vi "target - multi rate - variables - fileIO.vi"() -> ()   [LabVIEW 2011]
uses:
  Output - Cluster.ctl
  <vilib>/Platform/TimedLoop/XDataNode/timing_clust.ctl
  <vilib>/Platform/TimedLoop/XDataNode/nitl_modes.ctl
  <vilib>/Platform/TimedLoop/XDataNode/wakeup.ctl
  Input - Cluster.ctl
  <vilib>/functionblocks/Counter/Count Up/Count Up.vi
  <vilib>/functionblocks/Control/PID/PID.vi
  <vilib>/Platform/TimedLoop/XDataNode/XDataNode.xnode
  <vilib>/functionblocks/FB Core/FB Core.xnode
  <vilib>/functionblocks/FB Property/FB Overlay DBL.ctl
  <vilib>/Platform/TimedLoop/XDataNode/XDNodeRunTimeDep.lvlib
  <vilib>/functionblocks/NI_FunctionBlock Libraries.lvlib
panel:
  in  "shiftReg":T1
  in  "Output - Cluster":T2 {"TS-4" format="%#.2g"; "FS-2" format="%.2g"; "FS-1" format="%.2g"}
  # "The Network Variable Engine and Variable Client Support must be installed on the RT target\nfor this application to function properly. If the Network Variable Engine is not supported on\nthe target (e.g.  FP-2000 with <32MB of RAM), open the project and move the variable library\nto My Computer in the project. Doing this will deploy the variables to localhost but\nwill still require that Variable Client Support be installed on the RT target."
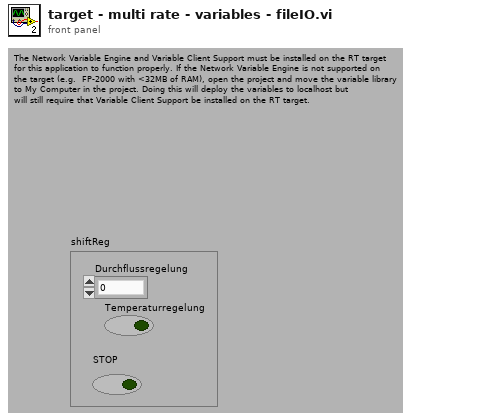
[diagram p1: front panel]
types:
  T1 = cluster{"Durchflussregelung":dbl, "Temperaturregelung":bool, "STOP":bool}
  T2 = typedef "Output - Cluster.ctl" = cluster{"DFS-1 Volumen":u64, "FS-3":dbl, "DFS-1 Durchfluss":dbl, "DS-1":dbl, "V-10 0":bool, "V-14 0":bool, "FS-1":dbl, "FS-2":dbl, "TS-4":dbl, "HS-1":bool, "V-13":u8, "V-15":u8, "P-4 Drehzahl":u8, "P-5 Drehzahl":u8, "Dosierung":bool, "MR Max Füllstand":bool, "MR Min Füllstand":bool, "Dosiermenge":sgl, "V-14 1":bool, "V-10 1":bool, "T-1 Max Füllstand":bool, "T-1 Min Füllstand":bool, "T-2 Max Füllstand":bool, "T-2 Min Füllstand":bool}
  T3 = enum16{"open", "replace", "create", "open or create", "replace or create", "replace or create with confirmation"}
  T4 = typedef "XDNodeRunTimeDep.lvlib/timing_clust.ctl" = cluster{"Expected End [f-1]":u64, "Actual End [f-1]":u64, "Finished Late? [f-1]":bool, "Expected End [i-1]":u64, "Actual End [i-1]":u64, "Finished Late? [i-1]":bool, "Expected Start [i]":u64, "Actual Start [i]":u64, "Expected Start [f]":u64, "Actual Start [f]":u64, "Source Name":string, "Structure Name":string, "Period":i64, "Deadline":i64, "Offset":i64, "Start":i64, "Priority":i32, "Timeout":i32, "Mode":T5, "Wakeup Reason":T6, "Error":errorcluster, "Source Type":string, "Secondary Source Type":string, "Global End Time":u64, "Global Start Time":u64, "Frame Duration":u64, "Iteration Duration":u64, "Assigned CPU":i32, "I/O Scan Engine Mode":u32}
  T5 = typedef "XDNodeRunTimeDep.lvlib/nitl_modes.ctl" = enum32{"No Change", "Process missed periods, maintain original phase", "Discard missed periods, maintain original phase", "Process missed periods, ignore original phase", "Discard missed periods, ignore original phase"}
  T6 = typedef "XDNodeRunTimeDep.lvlib/wakeup.ctl" = enum32{"Normal", "Aborted", "Asynchronous wakeup", "Timing source error", "Timed loop error", "Timeout"}
  T7 = typedef "Input - Cluster.ctl" = cluster{"V-13":u8, "V-15":u8, "Log-Target":bool, "P-4":bool, "P-4 Drehzahl [%]":u8, "Temperaturregelung":bool, "Überdruckregelung":bool, "Füllstandsregulierung":bool, "V-10":bool, "Log-Host":bool, "V-14":bool, "P-5":bool, "P-5 Drehzahl [%]":u8, "HS-1":bool, "Füllstand  P":sgl, "Füllstand I":sgl, "Füllstand D":sgl, "Füllstand Soll [%]":sgl, "Druck  P":sgl, "Druck I":sgl, "Druck D":sgl, "Druck Soll [bar]":sgl, "Temp Soll [°C]":sgl, "Dosierung":bool, "Dosiermenge [l]":sgl, "Dosiergeschw. [l/min]":sgl, "Zulauf":bool, "Hysterese[°C]":sgl, "MR Füllstandsüberwachung":bool, "Zulauf Füllstandsüberwachung":bool}
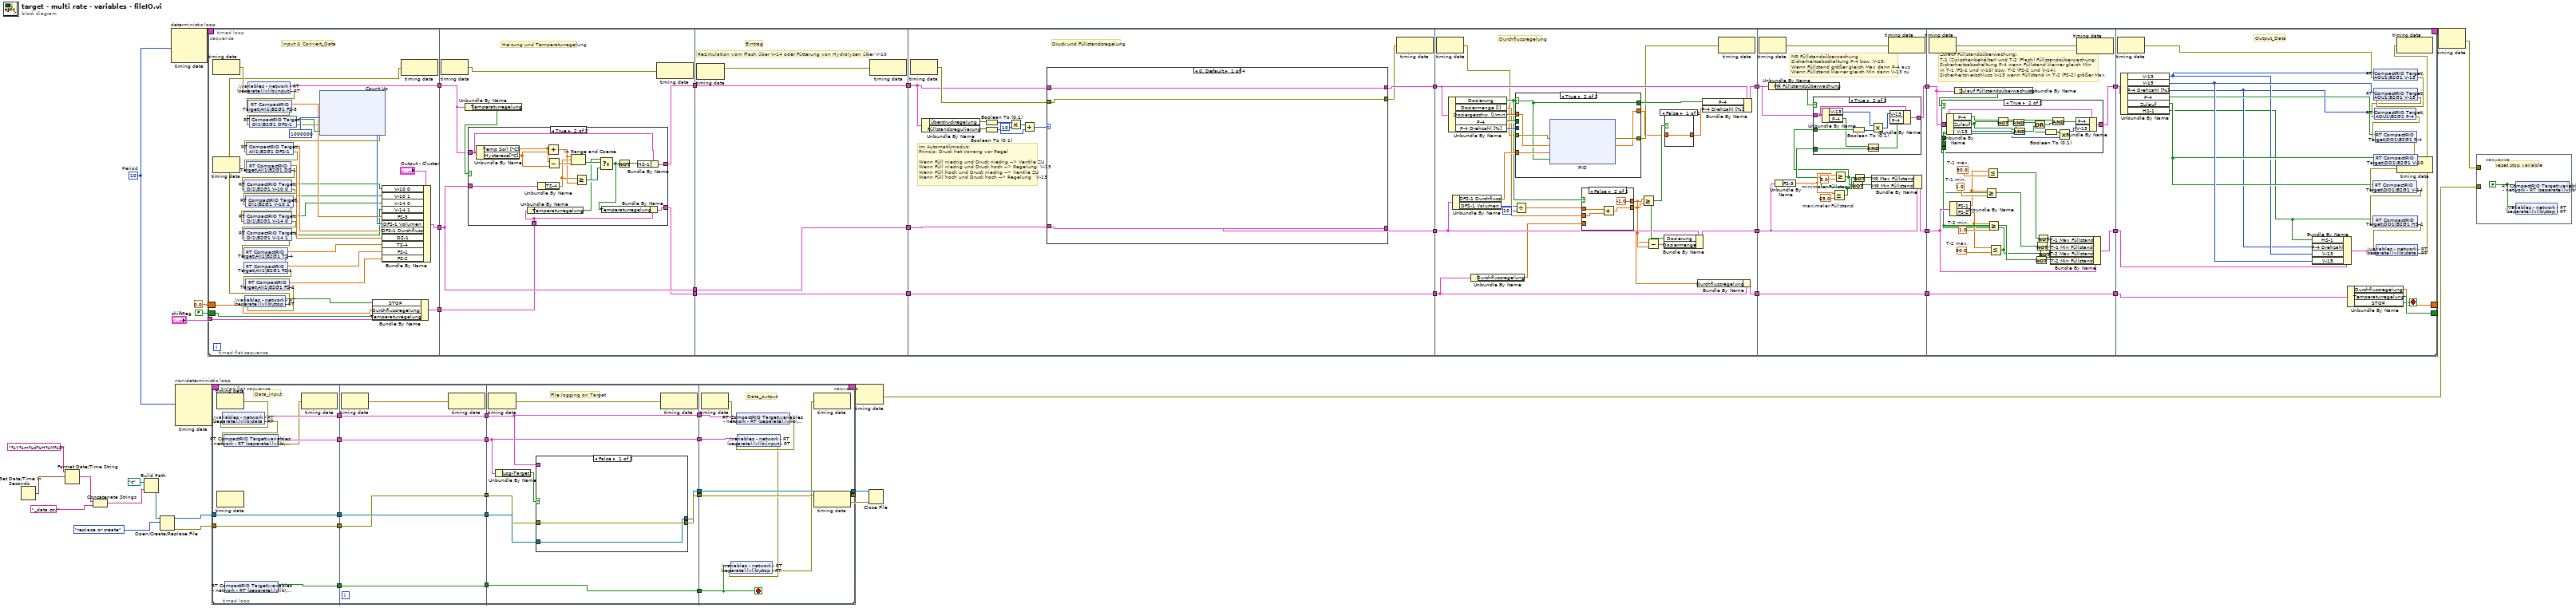
[diagram p0: block diagram]
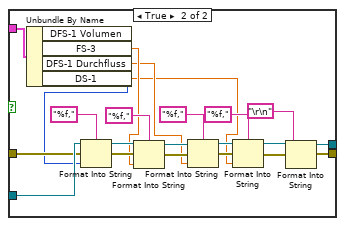
[diagram p2: hidden frame]
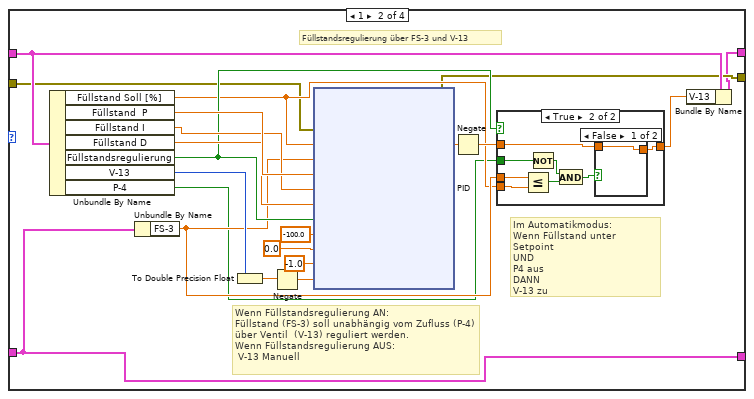
[diagram p4: hidden frame]
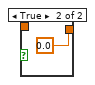
[diagram p6: hidden frame]
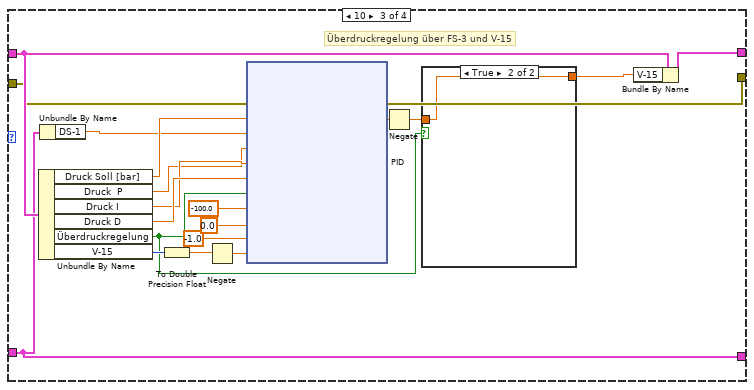
[diagram p7: hidden frame]
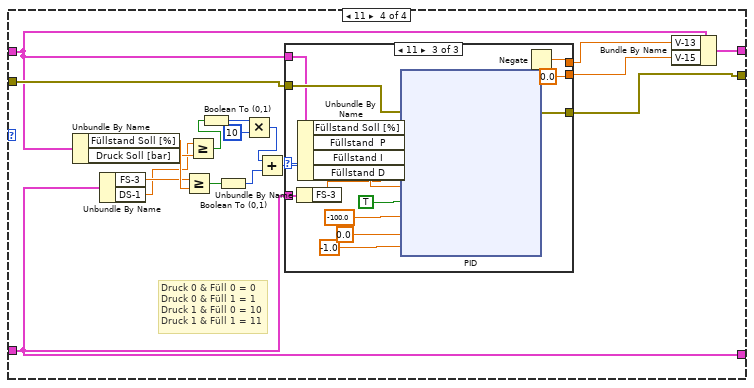
[diagram p9: hidden frame]
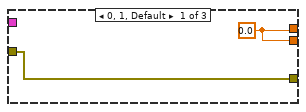
[diagram p10: hidden frame]
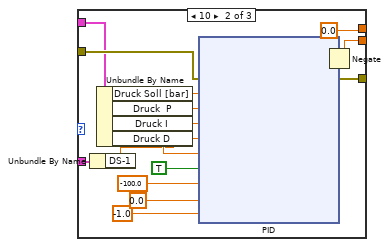
[diagram p11: hidden frame]
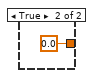
[diagram p13: hidden frame]
diagram:
  w15 = i64 10  # Period
  n1 = Get Date/Time In Seconds() -> (seconds since 1Jan1904=w11:timestamp)
  n2 = Format Date/Time String(time format string (%c)="%Y%m%d%H%M%S", seconds (now)=w11) -> (date/time string=w10:string)  [unwired: 1 in]
  n3 = Concatenate Strings(w10, "_data.csv" ("name or relative path")) -> (w7:string)
  n4 = Build Path(base path=path "c:/", name or relative path=w7) -> (appended path=w6:path)
  n5 = Open/Create/Replace File(file path (use dialog)=w6, operation (0:open)=T3."replace or create") -> (refnum out=w17:refnum<file>, error out=w16:errorcluster)  [unwired: 4 in, 1 out]
  n6 = node-c288 ("Input Node")(w15) -> (w22:T4)  [unwired: 2 in]
  n7 = node-c288 ("Input Node")(w15) -> (w20:T4)  [unwired: 3 in]
  n8 = timed-loop "deterministic loop" {
    timing: w22 -> [_]
    timing-out: [_] -> w21
    shift-right: [w27] -> _
    shift-left: 0.0 -> [w26]
    shift-right: [w25] -> _
    shift-left: FALSE ("Temperaturregelung") -> [w23]
    tunnel: "shiftReg" -> [w24]
    stop <- w759 stop-if-true
    n9 = timed-sequence {
      timing: _ -> [_]
      timing-out: _ -> [_]
      tunnel: [w51] -> w27
      tunnel: w26 -> [w50]
      tunnel: [w43] -> w25
      tunnel: w24 -> [w42]
      tunnel: w23 -> [w40]
      n10 = timed-flat-sequence {
        tunnel: [w87] -> w47
        tunnel: [w81] -> w45
        tunnel: w50 -> [w63]
        tunnel: w42 -> [w62]
        tunnel: [w61] -> w41
        tunnel: w40 -> [w60]
        tunnel: w47 -> [w140]
        tunnel: [w139] -> w46
        tunnel: w45 -> [w144]
        tunnel: [w144] -> w44
        tunnel: w41 -> [w143]
        tunnel: [w142] -> w39
        tunnel: w46 -> [w169]
        tunnel: [w169] -> w49
        tunnel: w44 -> [w171]
        tunnel: [w171] -> w48
        tunnel: w39 -> [w168]
        tunnel: [w168] -> w38
        tunnel: [w190] -> w53
        tunnel: w49 -> [w185]
        tunnel: w48 -> [w187]
        tunnel: [w186] -> w52
        tunnel: w38 -> [w177]
        tunnel: [w177] -> w37
        tunnel: w53 -> [w593]
        tunnel: [w591] -> w36
        tunnel: w52 -> [w592]
        tunnel: [w583] -> w35
        tunnel: w37 -> [w571]
        tunnel: [w573] -> w34
        tunnel: w36 -> [w683]
        tunnel: [w684] -> w33
        tunnel: w35 -> [w693]
        tunnel: [w689] -> w31
        tunnel: w34 -> [w695]
        tunnel: [w695] -> w29
        tunnel: w33 -> [w712]
        tunnel: [w727] -> w32
        tunnel: w31 -> [w726]
        tunnel: [w725] -> w30
        tunnel: w29 -> [w731]
        tunnel: [w731] -> w28
        tunnel: w32 -> [w770]
        tunnel: w30 -> [w768]
        tunnel: [w760] -> w51
        tunnel: [w761] -> w43
        tunnel: w28 -> [w762]
        frame #0 {
          # "Input & Convert_Data"
          n11 = node-c288 ("Output Node")() -> (w86:errorcluster)  [unwired: 1 in]
          n12 = shared-variable ".\\variables - network - RT (separate).lvlib\\input - RT"(error in=w86) -> (w87:T7, error out=w79:errorcluster)
          n13 = shared-variable "RT CompactRIO Target\\AII1\\B2G1 FS-3"(error in=w79) -> (w80:dbl, error out=w78:errorcluster)
          n14 = shared-variable "RT CompactRIO Target\\DI1\\B2G1 DFS-1"(error in=w78) -> (w89:bool, error out=w77:errorcluster)
          n15 = xnode "Count Up"("error in"=w77, "preset value"=1000000, "count up"=w89) -> ("error out"=w76:errorcluster, "counter value"=w84:u32)  [unwired: 1 in, 1 out]
          n16 = shared-variable "RT CompactRIO Target\\AII1\\B2G1 DFS-1"(error in=w76) -> (w83:dbl, error out=w75:errorcluster)
          n17 = shared-variable "RT CompactRIO Target\\AII1\\B2G1 DS-1"(error in=w75) -> (w82:dbl, error out=w73:errorcluster)
          n18 = shared-variable "RT CompactRIO Target\\DI1\\B2G1 V-10 0"(error in=w73) -> (w69:bool, error out=w72:errorcluster)
          n19 = shared-variable "RT CompactRIO Target\\DI1\\B2G1 V-10 1"(error in=w72) -> (w68:bool, error out=w71:errorcluster)
          n20 = shared-variable "RT CompactRIO Target\\DI1\\B2G1 V-14 0"(error in=w71) -> (w67:bool, error out=w70:errorcluster)
          n21 = shared-variable "RT CompactRIO Target\\DI1\\B2G1 V-14 1"(error in=w70) -> (w66:bool, error out=w65:errorcluster)
          n22 = shared-variable "RT CompactRIO Target\\AII1\\B2G1 TS-4"(error in=w65) -> (w64:dbl, error out=w56:errorcluster)
          n23 = shared-variable "RT CompactRIO Target\\AII1\\B2G1 FS-1"(error in=w56) -> (w58:dbl, error out=w55:errorcluster)
          n24 = shared-variable "RT CompactRIO Target\\AII1\\B2G1 FS-2"(error in=w55) -> (w57:dbl, error out=w54:errorcluster)
          n25 = shared-variable ".\\variables - network - RT (separate).lvlib\\stop - RT"(error in=w54) -> (w59:bool, error out=w74:errorcluster)
          n26 = Bundle By Name(cluster=w62, "STOP"=w59, "Durchflussregelung"=w63, "Temperaturregelung"=w60) -> (w61:T1)
          n27 = Bundle By Name(cluster="Output - Cluster", "V-10 0"=w69, "V-10 1"=w68, "V-14 0"=w67, "V-14 1"=w66, "FS-3"=w80, "DFS-1 Volumen"=w84, "DFS-1 Durchfluss"=w83, "DS-1"=w82, "TS-4"=w64, "FS-1"=w58, "FS-2"=w57) -> (w81:T2)
          n28 = node-c288 ("Input Node")(w74) -> ()  [unwired: 1 out]
        }
        frame #1 {
          # "Heizung und Temperaturregelung"
          n29 = node-c288() -> (w145:errorcluster)  [unwired: 1 in]
          n30 = Unbundle By Name(w140) -> ("Temperaturregelung"=w141:bool)
          n31 = case shown="True" w141 {
            tunnel: w144 -> [_ w157]
            tunnel: w143 -> [w147 w154]
            tunnel: [w147 w152] -> w142
            tunnel: w140 -> [w146 w148]
            tunnel: [w146 w150] -> w139
            frame False {
            }
            frame True {
              n32 = Unbundle By Name(w148) -> ("Temp Soll [°C]"=w158:sgl, "Hysterese[°C]"=w151:sgl)
              n33 = Unbundle By Name(w154) -> ("Temperaturregelung"=w155:bool)
              n34 = Unbundle By Name(w157) -> ("TS-4"=w156:dbl)
              n35 = Add(x=w158, y=w151) -> (x+y=w160:sgl)
              n36 = Subtract(x=w158, y=w151) -> (x-y=w162:sgl)
              n37 = In Range and Coerce(upper limit=w160, x=w156, lower limit=w162) -> (In Range?=w161:bool)  [unwired: 1 out]
              n38 = Greater Or Equal?(x=w156, y=w160) -> (x >= y?=w159:bool)
              n39 = Select(t=w155, s=w161, f=w159) -> (s? t:f=w153:bool)
              n40 = Bundle By Name(cluster=w154, "Temperaturregelung"=w153) -> (w152:T1)
              n41 = Not(x=w153) -> (.not. x?=w149:bool)
              n42 = Bundle By Name(cluster=w148, "HS-1"=w149) -> (w150:T7)
            }
          }
          n43 = node-c288(w145) -> ()  [unwired: 1 out]
        }
        frame #2 {
          # "Rezirkulation vom Flash über V-14 oder Fütterung von Hydrolysen über V-10"
          # "Eintrag"
          n44 = node-c288() -> (w170:errorcluster)  [unwired: 1 in]
          n45 = node-c288(w170) -> ()  [unwired: 1 out]
        }
        frame #3 {
          # "Im Automatikmodus:\nPrinzip: Druck hat Vorrang vor Pegel\n\nWenn Füll niedrig und Druck niedrig --> Ventile ZU\nWenn Füll niedrig und Druck hoch --> Regelung  V-15\nWenn Füll hoch und Druck niedrig --> Ventile ZU\nWenn Füll hoch und Druck hoch --> Regelung   V-13"
          # "Druck und Füllstandsregelung"
          n46 = node-c288() -> (w189:errorcluster)  [unwired: 1 in]
          n47 = Unbundle By Name(w185) -> ("Überdruckregelung"=w184:bool, "Füllstandsregulierung"=w183:bool)
          n48 = Boolean To (0,1)(Boolean=w183) -> (0, 1=w179:i16)
          n49 = Boolean To (0,1)(Boolean=w184) -> (0, 1=w182:i16)
          n50 = Multiply(x=w182, y=i16 10) -> (x*y=w180:i16)
          n51 = Add(x=w180, y=w179) -> (x+y=w178:i16)
          n52 = case shown="0, Default" w178 {
            tunnel: w185 -> [w193 w200 w311 w381]
            tunnel: [w193 w197 w310 w384] -> w190
            tunnel: w189 -> [w192 w199 w309 w382]
            tunnel: [w192 w198 w308 w383] -> w188
            tunnel: w187 -> [w191 w194 w292 w380]
            tunnel: [w191 w194 w292 w380] -> w186
            frame 0, Default {
            }
            frame 1 {
              # "Füllstandsregulierung über FS-3 und V-13"
              # "Wenn Füllstandsregulierung AN:\nFüllstand (FS-3) soll unabhängig vom Zufluss (P-4) \nüber Ventil  (V-13) reguliert werden.\nWenn Füllstandsregulierung AUS:\n V-13 Manuell"
              # "Im Automatikmodus:\nWenn Füllstand unter Setpoint\nUND\nP4 aus\nDANN\nV-13 zu"
              n53 = Unbundle By Name(w200) -> ("Füllstand Soll [%]"=w203:sgl, "Füllstand  P"=w214:sgl, "Füllstand I"=w213:sgl, "Füllstand D"=w212:sgl, "Füllstandsregulierung"=w207:bool, "V-13"=w208:u8, "P-4"=w202:bool)
              n54 = Unbundle By Name(w194) -> ("FS-3"=w204:dbl)
              n55 = To Double Precision Float(number=w208) -> (double precision float=w195:dbl)
              n56 = Negate(x=w195) -> (-x=w196:dbl)
              n57 = xnode "PID"("error in"=w199, "setpoint"=w203, "process variable"=w204, "proportional gain (Kc)"=w214, "integral time (Ti, min)"=w213, "derivative time (Td, min)"=w212, "auto? (T)"=w207, "output low"=-100.0, "output high"=0.0, "dt (s)"=-1.0, "manual control"=w196) -> ("error out"=w198:errorcluster, "output"=w211:dbl)
              n58 = Negate(x=w211) -> (-x=w205:dbl)
              n59 = case shown="True" w207 {
                tunnel: [w215 w218] -> w206
                tunnel: w205 -> [w215 w217]
                tunnel: w204 -> [_ w223]
                tunnel: w203 -> [_ w222]
                tunnel: w202 -> [_ w216]
                frame False {
                }
                frame True {
                  n60 = Less Or Equal?(x=w223, y=w222) -> (x <= y?=w221:bool)
                  n61 = Not(x=w216) -> (.not. x?=w220:bool)
                  n62 = And(x=w220, y=w221) -> (x .and. y?=w219:bool)
                  n63 = case shown="False" w219 {
                    tunnel: [w224 0.0] -> w218
                    tunnel: w217 -> [w224 _]
                    frame False {
                    }
                    frame True {
                    }
                  }
                }
              }
              n64 = Bundle By Name(cluster=w200, "V-13"=w206) -> (w197:T7)
            }
            frame 10 {
              # "Überdruckregelung über FS-3 und V-15"
              n65 = Unbundle By Name(w311) -> ("Druck Soll [bar]"=w299:sgl, "Druck  P"=w298:sgl, "Druck I"=w300:sgl, "Druck D"=w301:sgl, "Überdruckregelung"=w295:bool, "V-15"=w306:u8)
              n66 = Unbundle By Name(w292) -> ("DS-1"=w297:dbl)
              n67 = To Double Precision Float(number=w306) -> (double precision float=w305:dbl)
              n68 = Negate(x=w305) -> (-x=w307:dbl)
              n69 = xnode "PID"("error in"=w309, "setpoint"=w299, "process variable"=w297, "proportional gain (Kc)"=w298, "integral time (Ti, min)"=w300, "derivative time (Td, min)"=w301, "auto? (T)"=w295, "output low"=-100.0, "output high"=0.0, "dt (s)"=-1.0, "manual control"=w307) -> ("error out"=w308:errorcluster, "output"=w296:dbl)
              n70 = Negate(x=w296) -> (-x=w294:dbl)
              n71 = case shown="True" w295 {
                tunnel: [w312 w313] -> w293
                tunnel: w294 -> [w312 w313]
                frame False {
                }
                frame True {
                }
              }
              n72 = Bundle By Name(cluster=w311, "V-15"=w293) -> (w310:T7)
            }
            frame 11 {
              # "Druck 0 & Füll 0 = 0\nDruck 0 & Füll 1 = 1\nDruck 1 & Füll 0 = 10\nDruck 1 & Füll 1 = 11"
              n73 = Unbundle By Name(w381) -> ("Füllstand Soll [%]"=w397:sgl, "Druck Soll [bar]"=w391:sgl)
              n74 = Unbundle By Name(w380) -> ("FS-3"=w396:dbl, "DS-1"=w390:dbl)
              n75 = Greater Or Equal?(x=w396, y=w397) -> (x >= y?=w394:bool)
              n76 = Greater Or Equal?(x=w390, y=w391) -> (x >= y?=w395:bool)
              n77 = Boolean To (0,1)(Boolean=w395) -> (0, 1=w389:i16)
              n78 = Boolean To (0,1)(Boolean=w394) -> (0, 1=w393:i16)
              n79 = Multiply(x=w389, y=i16 10) -> (x*y=w387:i16)
              n80 = Add(x=w387, y=w393) -> (x+y=w392:i16)
              n81 = case shown="11" w392 {
                tunnel: [w399 0.0 ("V-13") w485] -> w386
                tunnel: [w399 w405 0.0 ("V-13")] -> w385
                tunnel: w382 -> [w398 w404 w489]
                tunnel: [w398 w407 w488] -> w383
                tunnel: w380 -> [_ w403 w484]
                tunnel: w381 -> [_ w402 w483]
                frame 0, 1, Default {
                  w399 = 0.0 ("V-13")
                }
                frame 10 {
                  n82 = Unbundle By Name(w403) -> ("DS-1"=w408:dbl)
                  n83 = Unbundle By Name(w402) -> ("Druck Soll [bar]"=w412:sgl, "Druck  P"=w411:sgl, "Druck I"=w410:sgl, "Druck D"=w409:sgl)
                  n84 = xnode "PID"("error in"=w404, "setpoint"=w412, "process variable"=w408, "proportional gain (Kc)"=w411, "integral time (Ti, min)"=w410, "derivative time (Td, min)"=w409, "auto? (T)"=TRUE, "output low"=-100.0, "output high"=0.0, "dt (s)"=-1.0) -> ("error out"=w407:errorcluster, "output"=w406:dbl)
                  n85 = Negate(x=w406) -> (-x=w405:dbl)
                }
                frame 11 {
                  n86 = Unbundle By Name(w484) -> ("FS-3"=w490:dbl)
                  n87 = Unbundle By Name(w483) -> ("Füllstand Soll [%]"=w494:sgl, "Füllstand  P"=w493:sgl, "Füllstand I"=w492:sgl, "Füllstand D"=w491:sgl)
                  n88 = xnode "PID"("error in"=w489, "setpoint"=w494, "process variable"=w490, "proportional gain (Kc)"=w493, "integral time (Ti, min)"=w492, "derivative time (Td, min)"=w491, "auto? (T)"=TRUE, "output low"=-100.0, "output high"=0.0, "dt (s)"=-1.0) -> ("error out"=w488:errorcluster, "output"=w486:dbl)
                  n89 = Negate(x=w486) -> (-x=w485:dbl)
                }
              }
              n90 = Bundle By Name(cluster=w381, "V-13"=w386, "V-15"=w385) -> (w384:T7)
            }
          }
          n91 = node-c288(w188) -> ()  [unwired: 1 out]
        }
        frame #4 {
          # "Durchflussregelung"
          n92 = node-c288() -> (w569:errorcluster)  [unwired: 1 in]
          n93 = Unbundle By Name(w593) -> ("Dosierung"=w579:bool, "Dosiermenge [l]"=w584:sgl, "Dosiergeschw. [l/min]"=w586:sgl, "P-4"=w589:bool, "P-4 Drehzahl [%]"=w588:u8)
          n94 = Unbundle By Name(w592) -> ("DFS-1 Durchfluss"=w585:dbl, "DFS-1 Volumen"=w577:u64)
          n95 = Unbundle By Name(w571) -> ("Durchflussregelung"=w570:dbl)
          n96 = Divide(x=w577, y=u64 10) -> (x/y=w576:dbl)
          n97 = case shown="True" w579 {
            selector: w579 -> [_ w605]
            tunnel: [w604 w605] -> w590
            tunnel: w589 -> [w604 _]
            tunnel: [w603 w608] -> w580
            tunnel: w588 -> [w603 _]
            tunnel: [w602 w610] -> w587
            tunnel: w569 -> [w602 w609]
            tunnel: w586 -> [_ w607]
            tunnel: w585 -> [_ w606]
            frame False {
            }
            frame True {
              n98 = xnode "PID"("error in"=w609, "setpoint"=w607, "process variable"=w606, "auto? (T)"=w605) -> ("error out"=w610:errorcluster, "output"=w608:dbl)
            }
          }
          n99 = case shown="False" w579 {
            tunnel: w584 -> [_ w598]
            tunnel: w576 -> [w594 w597]
            tunnel: [w595 w599] -> w572
            tunnel: w570 -> [w595 _]
            tunnel: [w594 -1.0] -> w574
            frame True {
            }
            frame False {
              n100 = Add(x=w597, y=w598) -> (x+y=w599:dbl)
            }
          }
          n101 = Greater Or Equal?(x=w574, y=w572) -> (x >= y?=w582:bool)
          n102 = Subtract(x=w572, y=w574) -> (x-y=w575:dbl)
          n103 = Bundle By Name(cluster=w592, "Dosierung"=w582, "Dosiermenge"=w575) -> (w583:T2)
          n104 = case shown="False" w582 {
            tunnel: [w600 0.0 ("output")] -> w581
            tunnel: w580 -> [w600 _]
            frame False {
            }
            frame True {
            }
          }
          n105 = Bundle By Name(cluster=w571, "Durchflussregelung"=w572) -> (w573:T1)
          n106 = Bundle By Name(cluster=w593, "P-4"=w590, "P-4 Drehzahl [%]"=w581) -> (w591:T7)
          n107 = node-c288(w587) -> ()  [unwired: 1 out]
        }
        frame #5 {
          w691 = 5.0  # minimaler Füllstand
          w692 = 65.0  # maximaler Füllstand
          # "MR Füllstandsüberwachung\nSicherheitsabschaltung P-4 bzw. V-13:\nWenn Füllstand größer gleich Max dann P-4 aus\nWenn Füllstand kleiner gleich Min dann V-13 zu"
          n108 = node-c288() -> (w694:errorcluster)  [unwired: 1 in]
          n109 = Unbundle By Name(w683) -> ("MR Füllstandsüberwachung"=w682:bool)
          n110 = Unbundle By Name(w693) -> ("FS-3"=w690:dbl)
          n111 = Less Or Equal?(x=w690, y=w692) -> (x <= y?=w688:bool)
          n112 = Greater Or Equal?(x=w690, y=w691) -> (x >= y?=w686:bool)
          n113 = case shown="True" w682 {
            tunnel: w688 -> [_ w704]
            tunnel: w686 -> [_ w703]
            tunnel: w683 -> [w696 w698]
            tunnel: [w696 w697] -> w684
            frame False {
            }
            frame True {
              n114 = Unbundle By Name(w698) -> ("V-13"=w702:u8, "P-4"=w701:bool)
              n115 = Boolean To (0,1)(Boolean=w703) -> (0, 1=w705:i16)
              n116 = And(x=w701, y=w704) -> (x .and. y?=w699:bool)
              n117 = Multiply(x=w702, y=w705) -> (x*y=w700:i16)
              n118 = Bundle By Name(cluster=w698, "V-13"=w700, "P-4"=w699) -> (w697:T7)
            }
          }
          n119 = Not(x=w686) -> (.not. x?=w685:bool)
          n120 = Not(x=w688) -> (.not. x?=w687:bool)
          n121 = Bundle By Name(cluster=w693, "MR Max Füllstand"=w687, "MR Min Füllstand"=w685) -> (w689:T2)
          n122 = node-c288(w694) -> ()  [unwired: 1 out]
        }
        frame #6 {
          w716 = 90.0  # T-1 max.
          w719 = 90.0  # T-2 max.
          w728 = 1.0  # T-2 min.
          w729 = 1.0  # T-1 min.
          # "Zulauf Füllstandsüberwachung:\nT-1 (Zwischenbehälter) und T-2 (Flash) Füllstandsüberwachung:\nSicherheitsabschaltung P-4 wenn Füllstand kleiner gleich Min\nin T-1 (FS-1 und V-10) bzw. T-2 (FS-2 und V-14).\nSicherheitsverschluss V-13 wenn Füllstand in T-2 (FS-2) größer Max."
          n123 = node-c288() -> (w730:errorcluster)  [unwired: 1 in]
          n124 = Unbundle By Name(w726) -> ("FS-1"=w715:dbl, "FS-2"=w720:dbl)
          n125 = Unbundle By Name(w712) -> ("Zulauf Füllstandsüberwachung"=w711:bool)
          n126 = Greater Or Equal?(x=w715, y=w729) -> (x >= y?=w723:bool)
          n127 = Less Or Equal?(x=w715, y=w716) -> (x <= y?=w714:bool)
          n128 = Greater Or Equal?(x=w720, y=w728) -> (x >= y?=w724:bool)
          n129 = Less Or Equal?(x=w720, y=w719) -> (x <= y?=w717:bool)
          n130 = case shown="True" w711 {
            tunnel: w712 -> [w732 w741]
            tunnel: [w732 w740] -> w727
            tunnel: w724 -> [_ w739]
            tunnel: w723 -> [_ w738]
            tunnel: w717 -> [_ w733]
            frame False {
            }
            frame True {
              n131 = Unbundle By Name(w741) -> ("P-4"=w743:bool, "Zulauf"=w746:bool, "V-13"=w737:u8)
              n132 = Not(x=w746) -> (.not. x?=w747:bool)
              n133 = And(x=w747, y=w738) -> (x .and. y?=w735:bool)
              n134 = And(x=w746, y=w739) -> (x .and. y?=w745:bool)
              n135 = Or(x=w735, y=w745) -> (x .or. y?=w744:bool)
              n136 = Boolean To (0,1)(Boolean=w733) -> (0, 1=w734:i16)
              n137 = And(x=w743, y=w744) -> (x .and. y?=w742:bool)
              n138 = Multiply(x=w734, y=w737) -> (x*y=w736:i16)
              n139 = Bundle By Name(cluster=w741, "P-4"=w742, "V-13"=w736) -> (w740:T7)
            }
          }
          n140 = Not(x=w724) -> (.not. x?=w721:bool)
          n141 = Not(x=w723) -> (.not. x?=w722:bool)
          n142 = Not(x=w714) -> (.not. x?=w713:bool)
          n143 = Not(x=w717) -> (.not. x?=w718:bool)
          n144 = Bundle By Name(cluster=w726, "T-1 Max Füllstand"=w713, "T-1 Min Füllstand"=w722, "T-2 Max Füllstand"=w718, "T-2 Min Füllstand"=w721) -> (w725:T2)
          n145 = node-c288(w730) -> ()  [unwired: 1 out]
        }
        frame #7 {
          # "Output_Data"
          n146 = node-c288() -> (w769:errorcluster)  [unwired: 1 in]
          n147 = Unbundle By Name(w770) -> ("V-13"=w755:u8, "V-15"=w766:u8, "P-4 Drehzahl [%]"=w754:u8, "P-4"=w756:bool, "Zulauf"=w763:bool, "HS-1"=w753:bool)
          n148 = Bundle By Name(cluster=w768, "HS-1"=w753, "P-4 Drehzahl"=w754, "V-13"=w755, "V-15"=w766) -> (w767:T2)
          n149 = Unbundle By Name(w762) -> ("Durchflussregelung"=w760:dbl, "Temperaturregelung"=w761:bool, "STOP"=w759:bool)
          n150 = shared-variable "RT CompactRIO Target\\AOU1\\B2G1 V-13"(w755, error in=w769) -> (error out=w774:errorcluster)
          n151 = shared-variable "RT CompactRIO Target\\AOU1\\B2G1 V-15"(w766, error in=w774) -> (error out=w773:errorcluster)
          n152 = shared-variable "RT CompactRIO Target\\AOU1\\B2G1 P-4"(w754, error in=w773) -> (error out=w772:errorcluster)
          n153 = shared-variable "RT CompactRIO Target\\DO1\\B2G1 P-4"(w756, error in=w772) -> (error out=w765:errorcluster)
          n154 = shared-variable "RT CompactRIO Target\\DO1\\B2G1 V-10"(w763, error in=w765) -> (error out=w764:errorcluster)
          n155 = shared-variable "RT CompactRIO Target\\DO1\\B2G1 V-14"(w763, error in=w764) -> (error out=w758:errorcluster)
          n156 = shared-variable "RT CompactRIO Target\\DO1\\B2G1 HS-1"(w753, error in=w758) -> (error out=w757:errorcluster)
          n157 = shared-variable ".\\variables - network - RT (separate).lvlib\\data - RT"(w767, error in=w757) -> (error out=w771:errorcluster)
          n158 = node-c288(w771) -> ()  [unwired: 1 out]
        }
      }
    }
    n159 = node-c288() -> ()  [unwired: 1 in, 1 out]
    n160 = node-c288() -> ()  [unwired: 1 in, 1 out]
  }
  n161 = timed-loop "non-deterministic loop" {
    timing: w20 -> [_]
    timing-out: [_] -> w19
    tunnel: w17 -> [w784]
    tunnel: w16 -> [w785]
    tunnel: [w783] -> w5
    tunnel: [w782] -> w4
    stop <- w873 stop-if-true
    n162 = timed-sequence {
      timing: _ -> [_]
      timing-out: _ -> [_]
      tunnel: w785 -> [w804]
      tunnel: w784 -> [w801]
      tunnel: [w799] -> w783
      tunnel: [w798] -> w782
      n163 = timed-flat-sequence {
        tunnel: w804 -> [w811]
        tunnel: w801 -> [w812]
        tunnel: [w812] -> w796
        tunnel: [w811] -> w795
        tunnel: [w810] -> w794
        tunnel: [w809] -> w793
        tunnel: [w808] -> w787
        tunnel: [w819] -> w803
        tunnel: [w823] -> w802
        tunnel: [w822] -> w800
        tunnel: [w820] -> w797
        tunnel: w796 -> [w823]
        tunnel: w795 -> [w822]
        tunnel: w794 -> [w820]
        tunnel: w793 -> [w819]
        tunnel: [w818] -> w788
        tunnel: w787 -> [w818]
        tunnel: w803 -> [w831]
        tunnel: w802 -> [w837]
        tunnel: w800 -> [w836]
        tunnel: w797 -> [w829]
        tunnel: [w835] -> w792
        tunnel: [w834] -> w791
        tunnel: [w831] -> w790
        tunnel: [w830] -> w789
        tunnel: w788 -> [w830]
        tunnel: [w829] -> w786
        tunnel: [w874] -> w798
        tunnel: [w875] -> w799
        tunnel: w792 -> [w875]
        tunnel: w791 -> [w874]
        tunnel: w790 -> [w873]
        tunnel: w789 -> [w872]
        tunnel: w786 -> [w871]
        frame #0 {
          # "Data_Input"
          n164 = node-c288() -> (w807:errorcluster)  [unwired: 1 in]
          n165 = shared-variable ".\\variables - network - RT (separate).lvlib\\data - RT"(error in=w807) -> (w810:T2, error out=w806:errorcluster)
          n166 = shared-variable "RT CompactRIO Target\\variables - network - RT (separate).lvlib\\input - network"(error in=w806) -> (w808:T7, error out=w805:errorcluster)
          n167 = shared-variable "RT CompactRIO Target\\variables - network - RT (separate).lvlib\\stop - network"() -> (w809:bool)  [unwired: 1 in, 1 out]
          n168 = node-c288(w805) -> ()  [unwired: 1 out]
        }
        frame #1 {
          n169 = node-c288 ("Output Node")() -> (w821:errorcluster)  [unwired: 1 in]
          n170 = node-c288(w821) -> ()  [unwired: 1 out]
        }
        frame #2 {
          # "File logging on Target"
          n171 = node-c288() -> (w833:errorcluster)  [unwired: 1 in]
          n172 = Unbundle By Name(w830) -> ("Log-Target"=w832:bool)
          n173 = case shown="False" w832 {
            tunnel: [w838 w861] -> w834
            tunnel: [w839 w860] -> w835
            tunnel: w837 -> [w838 w846]
            tunnel: w836 -> [w839 w845]
            tunnel: w829 -> [_ w844]
            frame False {
            }
            frame True {
              n174 = Unbundle By Name(w844) -> ("DFS-1 Volumen"=w843:u64, "FS-3"=w842:dbl, "DFS-1 Durchfluss"=w841:dbl, "DS-1"=w840:dbl)
              n175 = Format Into String(format string="%f,", initial string=w846, error in=w845, w843) -> (resulting string=w859:refnum<file>, error out=w856:errorcluster)
              n176 = Format Into String(format string="%f,", initial string=w859, error in=w856, w842) -> (resulting string=w858:refnum<file>, error out=w855:errorcluster)
              n177 = Format Into String(format string="%f,", initial string=w858, error in=w855, w841) -> (resulting string=w857:refnum<file>, error out=w854:errorcluster)
              n178 = Format Into String(format string="%f,", initial string=w857, error in=w854, w840) -> (resulting string=w848:refnum<file>, error out=w847:errorcluster)
              n179 = Format Into String(initial string=w848, error in=w847, "\r\n" ("input 1")) -> (resulting string=w861:refnum<file>, error out=w860:errorcluster)  [unwired: 1 in]
            }
          }
          n180 = node-c288(w833) -> ()  [unwired: 1 out]
        }
        frame #3 {
          # "Data_output"
          n181 = node-c288() -> (w870:errorcluster)  [unwired: 1 in]
          n182 = shared-variable "RT CompactRIO Target\\variables - network - RT (separate).lvlib\\data - network"(w871, error in=w870) -> (error out=w869:errorcluster)
          n183 = shared-variable ".\\variables - network - RT (separate).lvlib\\input - RT"(w872, error in=w869) -> (error out=w868:errorcluster)
          n184 = shared-variable ".\\variables - network - RT (separate).lvlib\\stop - RT"(w873, error in=w868) -> (error out=w867:errorcluster)
          n185 = node-c288(w867) -> ()  [unwired: 1 out]
        }
      }
    }
    n186 = node-c288() -> ()  [unwired: 1 in, 1 out]
    n187 = node-c288() -> ()  [unwired: 1 in, 1 out]
  }
  n188 = node-c288 ("Output Node")(w19) -> (w13:errorcluster)
  n189 = Close File(refnum=w4, error in=w5) -> ()  [unwired: 2 out]
  n190 = node-c288 ("Output Node")(w21) -> (w14:errorcluster)
  n191 = stacked-sequence {
    tunnel: w14 -> [_]
    tunnel: w13 -> [_]
    frame #0 {
      w883 = FALSE
      # "reset stop variable"
      n192 = shared-variable "RT CompactRIO Target\\variables - network - RT (separate).lvlib\\stop - network"(w883) -> ()  [unwired: 1 in, 1 out]
      n193 = shared-variable ".\\variables - network - RT (separate).lvlib\\stop - RT"(w883) -> ()  [unwired: 1 in, 1 out]
    }
  }
